vi "AquireRawPodsData.vi"(11 "All Pods In":T17(array[cluster])) -> (1 "Turret Angles":dbl[](array[numeric]), 2 "Drive Encoder Outputs":dbl[](array[numeric]), 3 "Pods States":T18(array[cluster]))   [LabVIEW 2014]
uses:
  <vilib>/Rock Robotics/WPI/MotorControl/WPI_MotorControlDeviceRef.ctl
  <vilib>/Rock Robotics/WPI/MotorControl/WPI_MotorControlType.ctl
  <vilib>/Rock Robotics/SystemInterfaces/Typedef/FPGA_TypedefDigitalModule.ctl
  <vilib>/Rock Robotics/SystemInterfaces/DIO/FPGA_DIOPWMChannel.ctl
  <vilib>/Rock Robotics/WPI/PWM/WPI_PWMDeadband.ctl
  <vilib>/Rock Robotics/WPI/CAN/Jaguar/SubVIs/WPI_CANJaguar_ControlMode.ctl
  <vilib>/Rock Robotics/WPI/CAN/TalonSRX/WPI_CANTalonSRX_APIControlMode.ctl
  <vilib>/Rock Robotics/WPI/PWM/WPI_PWMTransform_ConPane.ctl
  <vilib>/Rock Robotics/WPI/AnalogChannel/WPI_AnalogChannelDevRef.ctl
  <vilib>/Rock Robotics/SystemInterfaces/Typedef/FPGA_TypedefAnalogModule.ctl
  <vilib>/Rock Robotics/SystemInterfaces/AI/FPGA_AIChannel.ctl
  <vilib>/Rock Robotics/WPI/Encoder/WPI_EncoderDevRef.ctl
  <vilib>/Rock Robotics/SystemInterfaces/Encoder/FPGA_EncoderIdx.ctl
  <vilib>/Rock Robotics/SystemInterfaces/Counter/FPGA_CounterCtrSystemIndex.ctl
  <vilib>/Rock Robotics/WPI/Encoder/WPI_EncoderType.ctl
  Variables/References.vi
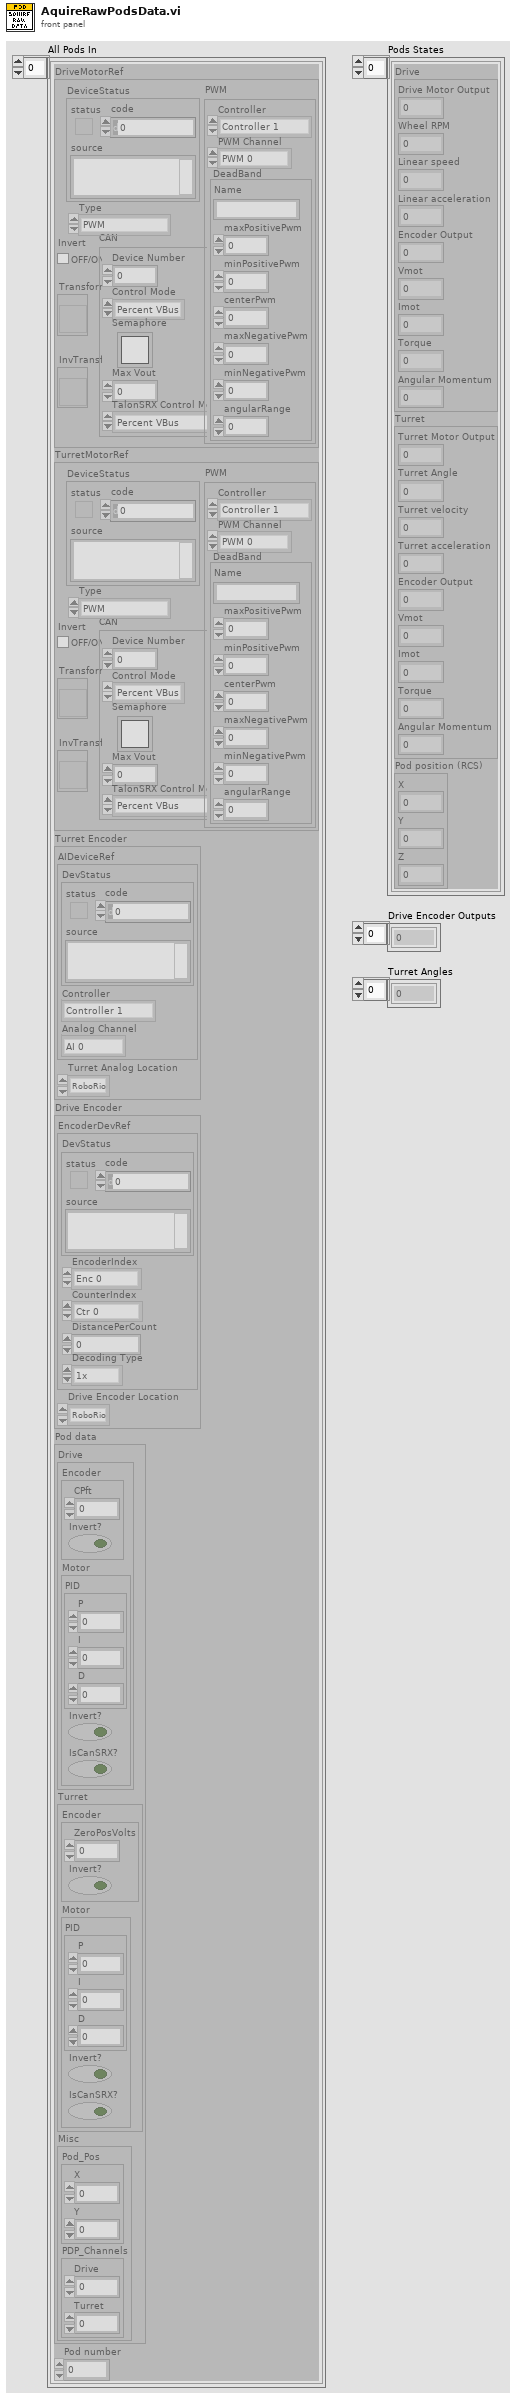
[diagram p1: front panel]
types:
  T1 = typedef "WPI_MotorControlDeviceRef.ctl" = cluster{"DeviceStatus":errorcluster, "Type":T2, "PWM":cluster{"Controller":T3, "PWM Channel":T4, "DeadBand":T5}, "CAN":cluster{"Device Number":u8, "Control Mode":T6, "Semaphore":T7, "Max Vout":dbl, "TalonSRX Control Mode":T8}, "Invert":bool, "TransformRef":T9, "InvTransformRef":T9}
  T2 = typedef "WPI_MotorControlType.ctl" = enum16{"PWM", "CAN", "CANTalonSRX"}
  T3 = typedef "FPGA_TypedefDigitalModule.ctl" = enum16{"Controller 1"}
  T4 = typedef "FPGA_DIOPWMChannel.ctl" = enum8{"PWM 0", "PWM 1", "PWM 2", "PWM 3", "PWM 4", "PWM 5", "PWM 6", "PWM 7", "PWM 8", "PWM 9", "PWM MXP 0", "PWM MXP 1", "PWM MXP 2", "PWM MXP 3", "PWM MXP 4", "PWM MXP 5", "PWM MXP 6", "PWM MXP 7", "PWM MXP 8", "PWM MXP 9", "Invalid"}
  T5 = typedef "WPI_PWMDeadband.ctl" = cluster{"Name":string, "maxPositivePwm":i32, "minPositivePwm":i32, "centerPwm":i32, "maxNegativePwm":i32, "minNegativePwm":i32, "angularRange":u16}
  T6 = typedef "WPI_CANJaguar_ControlMode.ctl" = enum8{"Percent VBus", "Current", "Speed", "Position", "Voltage"}
  T7 = typedef "Semaphore RefNum" = refnum<k1>
  T8 = typedef "WPI_CANTalonSRX_APIControlMode.ctl" = enum8{"Percent VBus", "Speed", "Position", "Slave", "Unchanged / Invalid"}
  T9 = typedef "WPI_PWMTransform_ConPane.ctl" = refnum<vi>
  T10 = typedef "WPI_AnalogChannelDevRef.ctl" = cluster{"DevStatus":errorcluster, "Controller":T11, "Analog Channel":T12}
  T11 = typedef "FPGA_TypedefAnalogModule.ctl" = enum16{"Controller 1"}
  T12 = typedef "FPGA_AIChannel.ctl" = enum8{"AI 0", "AI 1", "AI 2", "AI 3", "AI MXP 0", "AI MXP 1", "AI MXP 2", "AI MXP 3", "Invalid"}
  T13 = typedef "WPI_EncoderDevRef.ctl" = cluster{"DevStatus":errorcluster, "EncoderIndex":T14, "CounterIndex":T15, "DistancePerCount":dbl, "Decoding Type":T16}
  T14 = typedef "FPGA_EncoderIdx.ctl" = enum8{"Enc 0", "Enc 1", "Enc 2", "Enc 3", "Enc 4", "Enc 5", "Enc 6", "Enc 7", "Invalid"}
  T15 = typedef "FPGA_CounterCtrSystemIndex.ctl" = enum8{"Ctr 0", "Ctr 1", "Ctr 2", "Ctr 3", "Ctr 4", "Ctr 5", "Ctr 6", "Ctr 7", "Invalid"}
  T16 = typedef "WPI_EncoderType.ctl" = enum16{"1x", "2x", "4x"}
  T17 = cluster{"DriveMotorRef":T1, "TurretMotorRef":T1, "Turret Encoder":cluster{"AIDeviceRef":T10, "Turret Analog Location":enum16{"RoboRio", "Drive SRX", "Turret SRX"}}, "Drive Encoder":cluster{"EncoderDevRef":T13, "Drive Encoder Location":enum16{"RoboRio", "Drive SRX", "Turret SRX"}}, "Pod data":cluster{"Drive":cluster{"Encoder":cluster{"CPft":dbl, "Invert?":bool}, "Motor":cluster{"PID":cluster{"P":dbl, "I":dbl, "D":dbl}, "Invert?":bool, "IsCanSRX?":bool}}, "Turret":cluster{"Encoder":cluster{"ZeroPosVolts":dbl, "Invert?":bool}, "Motor":cluster{"PID":cluster{"P":dbl, "I":dbl, "D":dbl}, "Invert?":bool, "IsCanSRX?":bool}}, "Misc":cluster{"Pod_Pos":cluster{"X":dbl, "Y":dbl}, "PDP_Channels":cluster{"Drive":i32, "Turret":i32}}}, "Pod number":i32}[]
  T18 = cluster{"Drive":cluster{"Drive Motor Output":dbl, "Wheel RPM":dbl, "Linear speed":dbl, "Linear acceleration":dbl, "Encoder Output":dbl, "Vmot":dbl, "Imot":dbl, "Torque":dbl, "Angular Momentum":dbl}, "Turret":cluster{"Turret Motor Output":dbl, "Turret Angle":dbl, "Turret velocity":dbl, "Turret acceleration":dbl, "Encoder Output":dbl, "Vmot":dbl, "Imot":dbl, "Torque":dbl, "Angular Momentum":dbl}, "Pod position (RCS)":cluster{"X":dbl, "Y":dbl, "Z":dbl}}[]
  T19 = cluster{"Drive":cluster{"Drive Motor Output":dbl, "Wheel RPM":dbl, "Linear speed":dbl, "Linear acceleration":dbl, "Encoder Output":dbl, "Vmot":dbl, "Imot":dbl, "Torque":dbl, "Angular Momentum":dbl}, "Turret":cluster{"Turret Motor Output":dbl, "Turret Angle":dbl, "Turret velocity":dbl, "Turret acceleration":dbl, "Encoder Output":dbl, "Vmot":dbl, "Imot":dbl, "Torque":dbl, "Angular Momentum":dbl}, "Pod position (RCS)":cluster{"X":dbl, "Y":dbl, "Z":dbl}}
  T20 = typedef "WPI_CANTalonSRX_GlobalStatus.ctl" = cluster{"Applied Throttle":dbl, "Module Enabled":bool, "CAN Error":errorcluster, "Closed Loop Error":dbl, "Forward Limit Switch Closed":bool, "Reverse Limit Switch Closed":bool, "Sensor Position":dbl, "Sensor Velocity":dbl, "Current":dbl, "Sticky Fault - Over Temp":bool, "Sticky Fault - Under Voltage":bool, "Sticky Fault - Forward Limit":bool, "Sticky Fault - Reverse Limit":bool, "Sticky Fault - Forward Soft Limit":bool, "Sticky Fault - Reverse Soft Limit":bool, "Brake is Enabled":bool, "Encoder Position":dbl, "Encoder Velocity":dbl, "Encoder Index Count":dbl, "Encoder A Pin State":bool, "Encoder B Pin State":bool, "Encoder Index Pin State":bool, "Analog In":dbl, "Analog In Velocity":dbl, "Temperature (C)":dbl, "Battery Voltage":dbl}
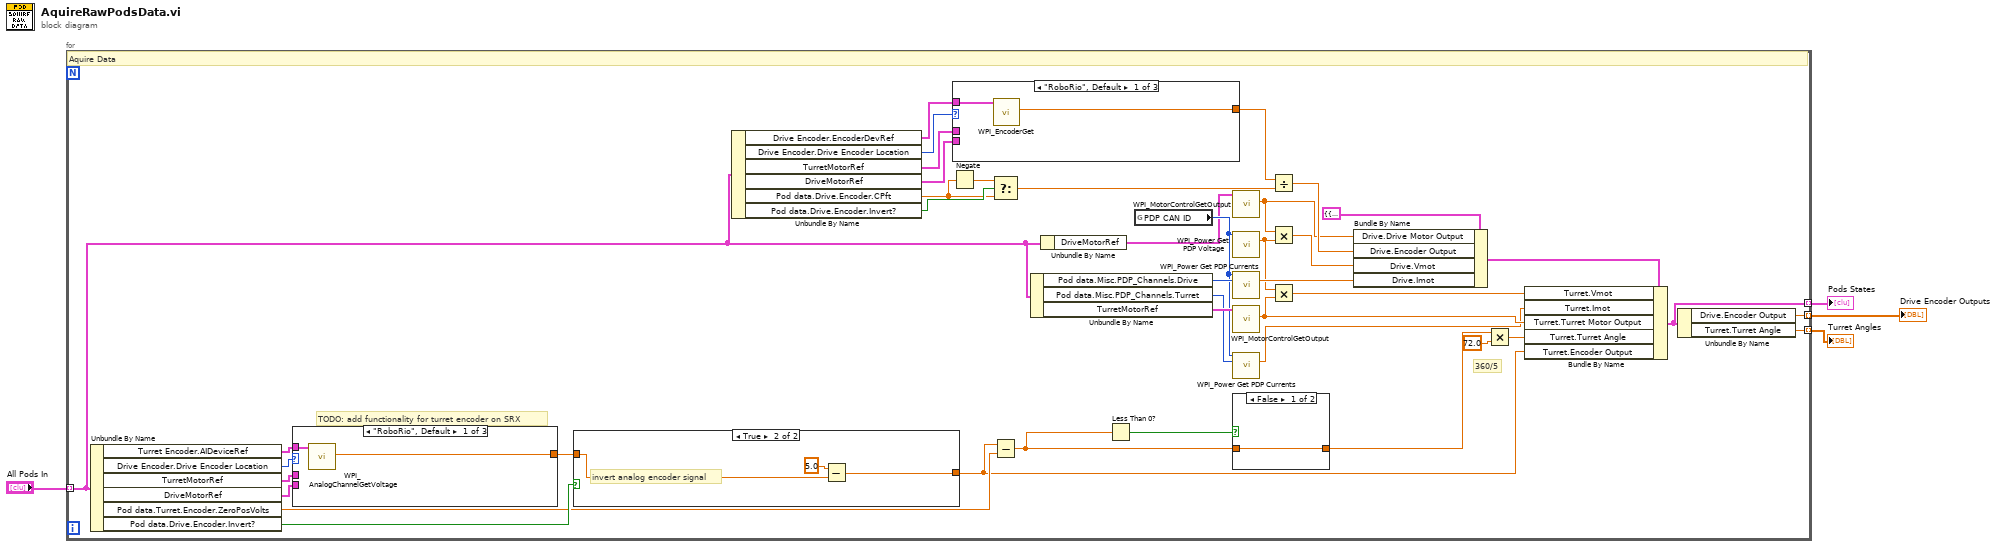
[diagram p0: block diagram]
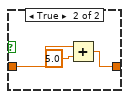
[diagram p2: hidden frame]
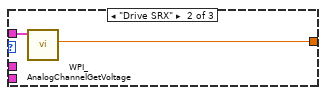
[diagram p4: hidden frame]
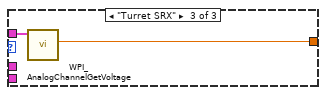
[diagram p5: hidden frame]
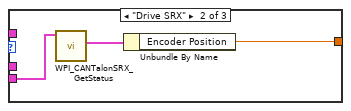
[diagram p6: hidden frame]
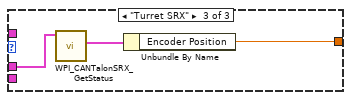
[diagram p7: hidden frame]
diagram:
  n1 = for {
    tunnel: "All Pods In" -> [w33] mode=indexing
    tunnel: [w19] -> w4 mode=indexing
    tunnel: [w18] -> w3 mode=indexing
    tunnel: [w17] -> w2 mode=indexing
    # "360/5"
    # "TODO: add functionality for turret encoder on SRX"
    # "Aquire Data"
    n2 = Unbundle By Name(w33) -> ("Turret Encoder.AIDeviceRef"=w35:T10, "Drive Encoder.Drive Encoder Location"=w34:enum16{"RoboRio", "Drive SRX", "Turret SRX"}, "TurretMotorRef"=w37:T1, "DriveMotorRef"=w36:T1, "Pod data.Turret.Encoder.ZeroPosVolts"=w29:dbl, "Pod data.Drive.Encoder.Invert?"=w31:bool)
    n3 = case shown="\"RoboRio\", Default" w34 {
      tunnel: w35 -> [w55 w57 w59]
      tunnel: w36 -> [_ _ _]
      tunnel: w37 -> [_ _ _]
      tunnel: [w54 w56 w58] -> w30
      frame "RoboRio", Default {
        n4 = call <vilib>:"WPI_AnalogChannelGetVoltage.vi"("AIDeviceRef"=w55) -> ("Voltage"=w54:dbl)  [unwired: 8 in, 2 out]
      }
      frame "Drive SRX" {
        n5 = call <vilib>:"WPI_AnalogChannelGetVoltage.vi"("AIDeviceRef"=w57) -> ("Voltage"=w56:dbl)  [unwired: 8 in, 2 out]
      }
      frame "Turret SRX" {
        n6 = call <vilib>:"WPI_AnalogChannelGetVoltage.vi"("AIDeviceRef"=w59) -> ("Voltage"=w58:dbl)  [unwired: 8 in, 2 out]
      }
    }
    n7 = case shown="True" w31 {
      tunnel: w30 -> [w50 w53]
      tunnel: [w50 w51] -> w20
      frame False {
      }
      frame True {
        # "invert analog encoder signal"
        n8 = Subtract(x=5.0, y=w53) -> (x-y=w51:dbl)
      }
    }
    n9 = Unbundle By Name(w33) -> ("Drive Encoder.EncoderDevRef"=w44:T13, "Drive Encoder.Drive Encoder Location"=w45:enum16{"RoboRio", "Drive SRX", "Turret SRX"}, "TurretMotorRef"=w42:T1, "DriveMotorRef"=w43:T1, "Pod data.Drive.Encoder.CPft"=w38:dbl, "Pod data.Drive.Encoder.Invert?"=w40:bool)
    n10 = Negate(x=w38) -> (-x=w39:dbl)
    n11 = case shown="\"RoboRio\", Default" w45 {
      tunnel: w44 -> [w61 _ _]
      tunnel: [w60 w62 w66] -> w23
      tunnel: w43 -> [_ w64 _]
      tunnel: w42 -> [_ _ w65]
      frame "RoboRio", Default {
        n12 = call <vilib>:"WPI_EncoderGet.vi"("EncoderDevRef"=w61) -> ("Distance"=w60:dbl)  [unwired: 5 in, 5 out]
      }
      frame "Drive SRX" {
        n13 = call <vilib>:"WPI_CANTalonSRX_GetStatus.vi"("CAN Talon SRX Ref"=w64) -> ("Talon SRX Status"=w63:T20)  [unwired: 8 in, 2 out]
        n14 = Unbundle By Name(w63) -> ("Encoder Position"=w62:dbl)
      }
      frame "Turret SRX" {
        n15 = call <vilib>:"WPI_CANTalonSRX_GetStatus.vi"("CAN Talon SRX Ref"=w65) -> ("Talon SRX Status"=w67:T20)  [unwired: 8 in, 2 out]
        n16 = Unbundle By Name(w67) -> ("Encoder Position"=w66:dbl)
      }
    }
    n17 = Select(t=w39, s=w40, f=w38) -> (s? t:f=w41:dbl)
    n18 = Subtract(x=w20, y=w29) -> (x-y=w25:dbl)
    n19 = Unbundle By Name(w33) -> ("Pod data.Misc.PDP_Channels.Drive"=w10:i32, "Pod data.Misc.PDP_Channels.Turret"=w8:i32, "TurretMotorRef"=w27:T1)
    n20 = Unbundle By Name(w33) -> ("DriveMotorRef"=w5:T1)
    n21 = Less Than 0?(x=w25) -> (x < 0?=w26:bool)
    n22 = global read "References.vi" "PDP CAN ID"() -> (w9:i32)
    n23 = call <vilib>:"WPI_MotorControlGetOutput.vi"("MotorControlDevRef"=w5) -> ("Output"=w16:dbl)  [unwired: 8 in, 2 out]
    n24 = call <vilib>:"WPI_Power Get PDP Voltage.vi"("Power Distribution Panel (0)"=w9) -> ("voltage (V)"=w12:dbl)  [unwired: 13 in, 1 out]
    n25 = call <vilib>:"WPI_Power Get PDP Currents.vi"("Power Distribution Panel (0)"=w9, "PDP Channel"=w10) -> ("current (A)"=w14:dbl)  [unwired: 11 in, 2 out]
    n26 = call <vilib>:"WPI_MotorControlGetOutput.vi"("MotorControlDevRef"=w27) -> ("Output"=w13:dbl)  [unwired: 8 in, 2 out]
    n27 = call <vilib>:"WPI_Power Get PDP Currents.vi"("Power Distribution Panel (0)"=w9, "PDP Channel"=w8) -> ("current (A)"=w7:dbl)  [unwired: 11 in, 2 out]
    n28 = case shown="False" w26 {
      tunnel: w25 -> [w46 w49]
      tunnel: [w46 w47] -> w24
      frame False {
      }
      frame True {
        n29 = Add(x=w49, y=5.0) -> (x+y=w47:dbl)
      }
    }
    n30 = Divide(x=w23, y=w41) -> (x/y=w21:dbl)
    n31 = Multiply(x=w16, y=w12) -> (x*y=w15:dbl)
    n32 = Multiply(x=w12, y=w13) -> (x*y=w11:dbl)
    n33 = Bundle By Name(cluster=T19 {"Drive"={"Drive Motor Output"=-1.0, "Wheel RPM"=0.0, "Linear speed"=0.0, "Linear acceleration"=0.0, "Encoder Output"=3.9794922919999998, "Vmot"=-12.950000000000001, "Imot"=0.0, "Torque"=0.0, "Angular Momentum"=0.0}, "Turret"={"Turret Motor Output"=0.0, "Turret Angle"=326.627445024, "Turret velocity"=0.0, "Turret acceleration"=0.0, "Encoder Output"=4.53613286, "Vmot"=0.0, "Imot"=0.0, "Torque"=0.0, "Angular Momentum"=0.0}, "Pod position (RCS)"={"X"=0.0, "Y"=0.0, "Z"=0.0}} ("element"), "Drive.Drive Motor Output"=w16, "Drive.Encoder Output"=w21, "Drive.Vmot"=w15, "Drive.Imot"=w14) -> (w32:T19)
    n34 = Multiply(x=w24, y=72.0) -> (x*y=w22:dbl)
    n35 = Bundle By Name(cluster=w32, "Turret.Vmot"=w11, "Turret.Imot"=w7, "Turret.Turret Motor Output"=w13, "Turret.Turret Angle"=w22, "Turret.Encoder Output"=w20) -> (w19:T19)
    n36 = Unbundle By Name(w19) -> ("Drive.Encoder Output"=w18:dbl, "Turret.Turret Angle"=w17:dbl)
  }
  "Pods States" <- w4
  "Drive Encoder Outputs" <- w3
  "Turret Angles" <- w2
